vi "Elliptic Filter PtByPt.vi"(0 "x":dbl format="%0.2f", 1 "passband ripple (dB)":dbl=1.0 format="%0.2f", 2 "filter type":T1, 3 "initialize":bool, 5 "sampling freq: fs":dbl=1.0 format="%0.2f", 9 "high cutoff freq: fh":dbl=0.45000000000000007 format="%0.3f", 11 "low cutoff freq: fl":dbl=0.125 format="%0.3f", 12 "stopband attenuation(dB)":dbl=60.0 format="%0.2f", 13 "order":i32=2) -> (4 "Filtered x":dbl format="%0.2f", 15 "error":i32)   [LabVIEW 2020, in "NI_PtbyPt.lvlib"]
doc: "Generates a digital elliptic filter by calling the Elliptic Coefficients VI."
uses:
  NI_PtbyPt.lvlib
  Filter Passband Type.ctl
  NI_AALBase.lvlib
panel:
  # "Filter Controls"
  # "Frequency Controls"
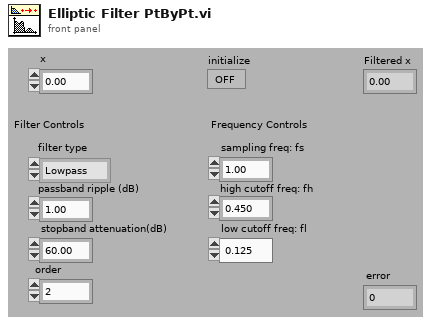
[diagram p1: front panel]
types:
  T1 = typedef "NI_AALBase.lvlib/Filter Passband Type.ctl" = enum32{"Lowpass", "Highpass", "Bandpass", "Bandstop"}
  T2 = cluster{"filter structure":enum32{"IIR 2nd Order", "IIR 4th Order"}, "Reverse Coefficients":dbl[], "Forward Coefficients":dbl[]}
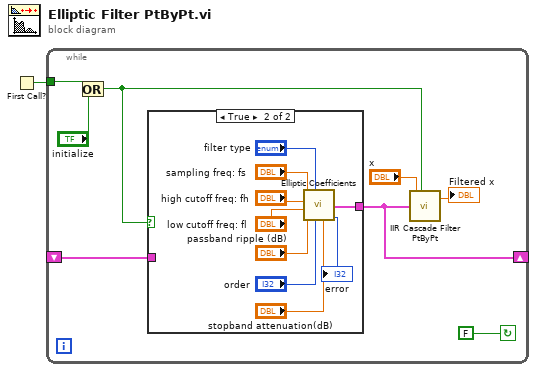
[diagram p0: block diagram]
diagram:
  n1 = First Call?() -> (First Call?: T/F=w1:bool)
  n2 = while {
    tunnel: w1 -> [w4]
    shift-left: _ -> [w8]
    shift-right: [w7] -> _
    stop <- FALSE continue-if-true
    n3 = Or(x=w4, y="initialize") -> (x .or. y?=w2:bool)
    n4 = case shown="True" w2 {
      tunnel: [w10 w19] -> w7
      tunnel: w8 -> [w10 _]
      frame False {
      }
      frame True {
        n5 = call "Elliptic Coefficients.vi"("stopband attenuation (dB)"="stopband attenuation(dB)", "order"="order", "filter type"="filter type", "passband ripple (dB)"="passband ripple (dB)", "low cutoff freq: fl"="low cutoff freq: fl", "high cutoff freq: fh"="high cutoff freq: fh", "sampling freq: fs"="sampling freq: fs") -> ("error"=→"error":i32, "IIR Filter Cluster"=w19:T2)  [unwired: 3 in]
      }
    }
    n6 = call "IIR Cascade Filter PtByPt.vi"("initialize"=w2, "IIR Filter Cluster"=w7, "x"="x") -> ("Filtered x"=→"Filtered x":dbl)  [unwired: 2 out]
  }
